vi "Pololu.Convert Low and Hi Bytes to Value.vi"(11 "Low_Hi Bytes":u8[](array[numeric]) format="%x") -> (3 "Value":u16)   [LabVIEW 2018, in "PololuCtrl.lvclass"]
uses:
  PololuCtrl.lvclass
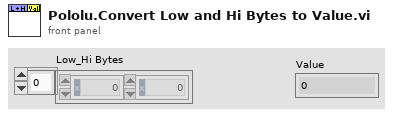
[diagram p1: front panel]
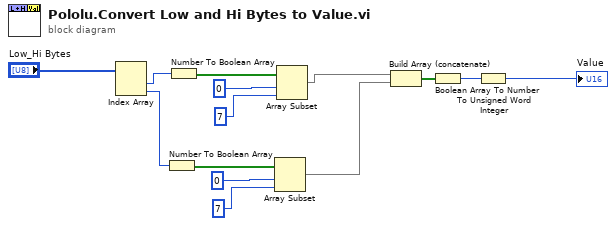
[diagram p0: block diagram]
diagram:
  n1 = Index Array(array="Low_Hi Bytes") -> (element #1=w10:u8, element #2=w6:u8)  [unwired: 2 in]
  n2 = Number To Boolean Array(number=w6) -> (Boolean array=w9:bool[])
  n3 = Number To Boolean Array(number=w10) -> (Boolean array=w12:bool[])
  n4 = Array Subset(array=w9, index=0, length=7) -> (w4:bool[])
  n5 = Array Subset(array=w12, index=0, length=7) -> (w5:bool[])
  n6 = Build Array (concatenate)(w5, w4) -> (w2:bool[])
  n7 = Boolean Array To Number(Boolean array=w2) -> (number=w3:u32)
  n8 = To Unsigned Word Integer(number=w3) -> (unsigned 16bit integer=→"Value":u16)
